vi "Untitled 1.vi"() -> ()   [LabVIEW 2025]
uses:
  <vilib>/LabVIEW Interface for Arduino/Type Defs/Pin Mode.ctl
  <vilib>/LabVIEW Interface for Arduino/LabVIEW Interface for Arduino.lvlib
panel:
  in  "stop":bool
  out "error out":errorcluster
  in  "Board":refnum<visa-resource-name>
  in  "Test cases":T1(ring)
  in  "Tab Control":T2(tab)
  in  "pin":u8
  in  "input val":u8
  out "Value":u8
  out "Outputs":bool[](array[boolean])
  in  "Set values":bool[](array[boolean])
  out "Voltage":dbl(knob) scale=0.0..5.0
  in  "Analog Input Pin (0)":u8
  out "Analog Port":dbl[](array[numeric])
  out "Waveform Chart":dbl(graph)
  in  "PWM 0 (0-255)":u8
  in  "PWM 1 (0-255)":u8
  in  "PWM 2 (0-255)":u8
  in  "PWM Pins":u8[](array[numeric])
  in  "Analog Input Pin":u8
  in  "pwm write single":u8
  in  "PWM Pin single":u8=3
  # "Arduino v4 tests"
  # "0x00 and 0x01 definitely work since every other case requires init and close to function"
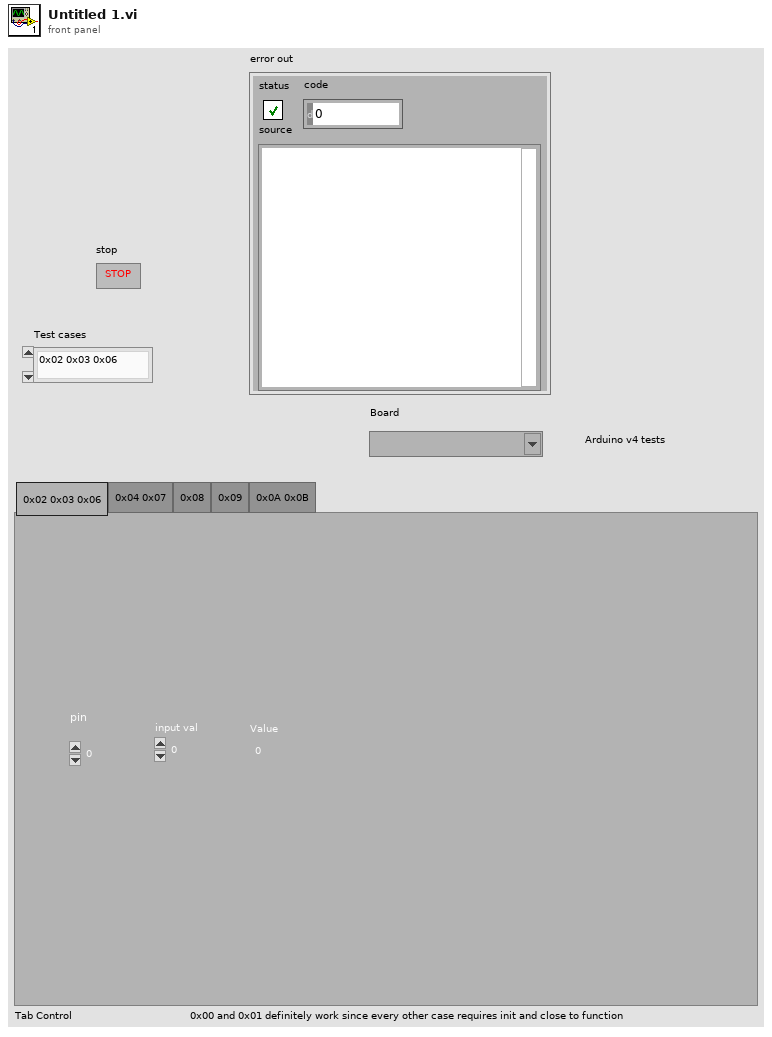
[diagram p1: front panel]
types:
  T1 = enum16{"0x02 0x03 0x06", "0x04 0x07", "0x08", "0x09", "0x0A 0x0B"}
  T2 = enum32{"0x02 0x03 0x06", "0x04 0x07", "0x08", "0x09", "0x0A 0x0B"}
  T3 = typedef "LabVIEW Interface for Arduino.lvlib/Pin Mode.ctl" = enum8{"Input", "Output"}
  T4 = typedef "LabVIEW Interface for Arduino.lvlib/Arduino Resource.ctl" = cluster{"VISA resource":refnum<visa-resource-name>, "Board Type":T5, "Connection Type":enum8{"USB / Serial"}, "Bytes Per Packet (15)":u8}
  T5 = typedef "LabVIEW Interface for Arduino.lvlib/Board Type.ctl" = enum16{"Uno", "Dimuelanove w/Atmega 328", "Mega 2560"}
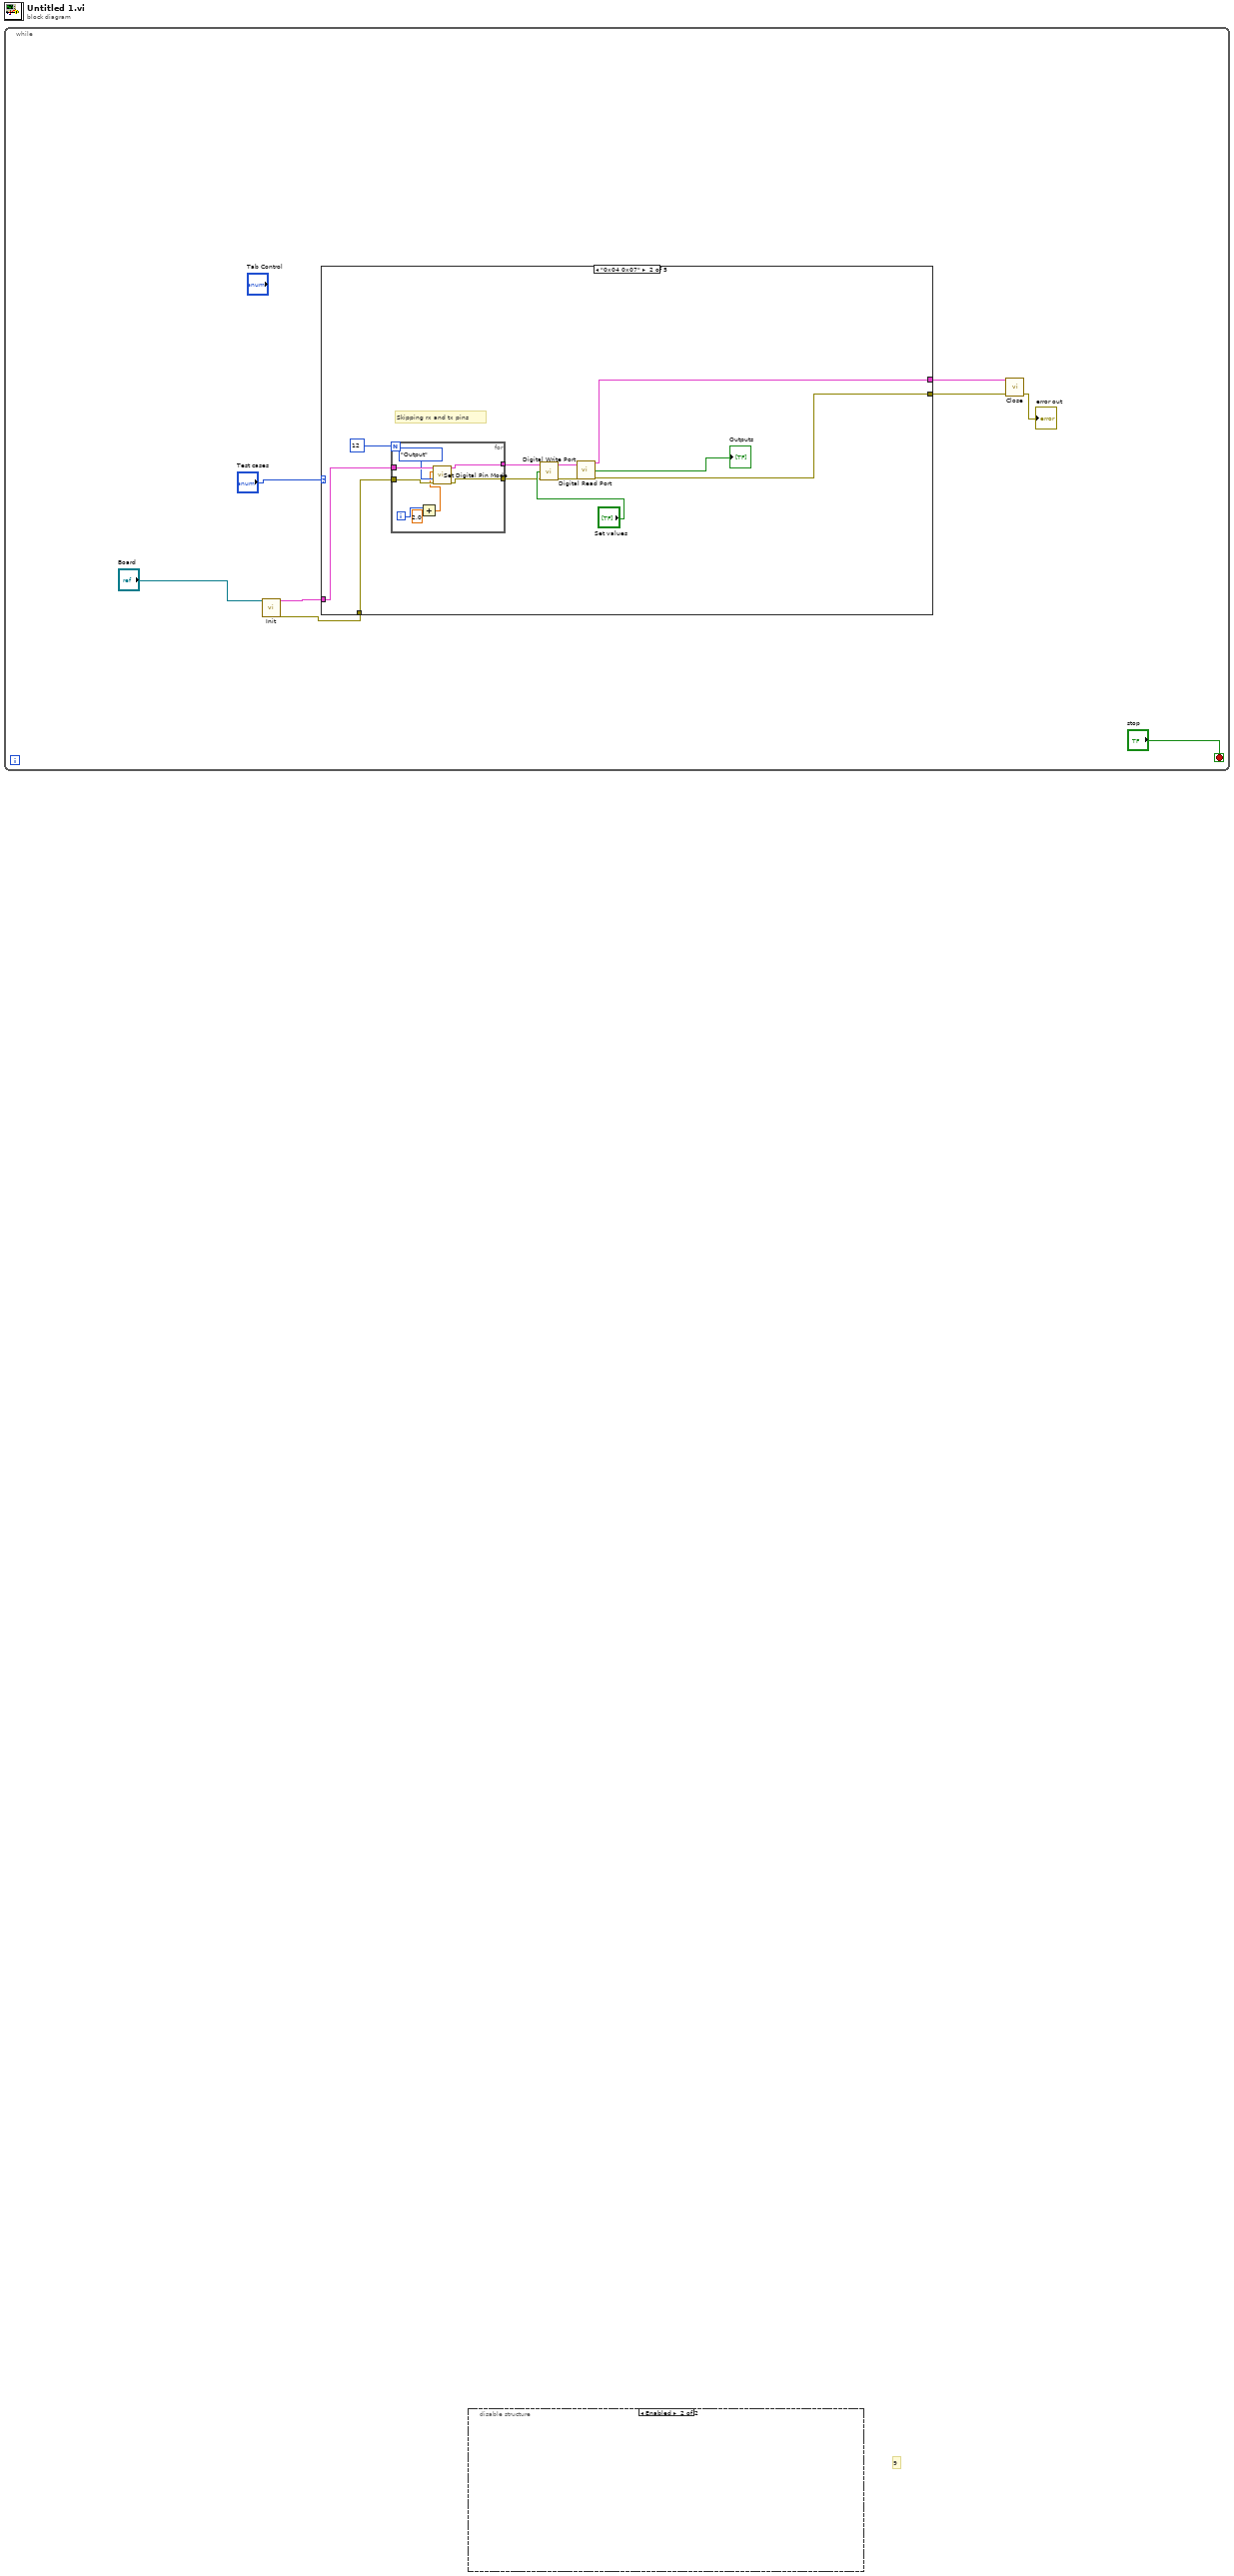
[diagram p0: block diagram]
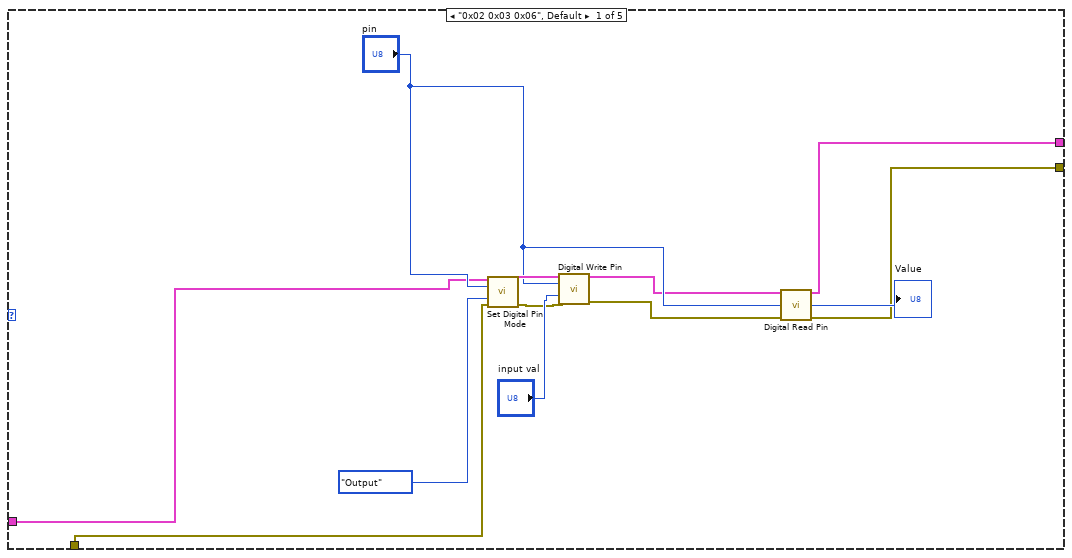
[diagram p2: hidden frame]
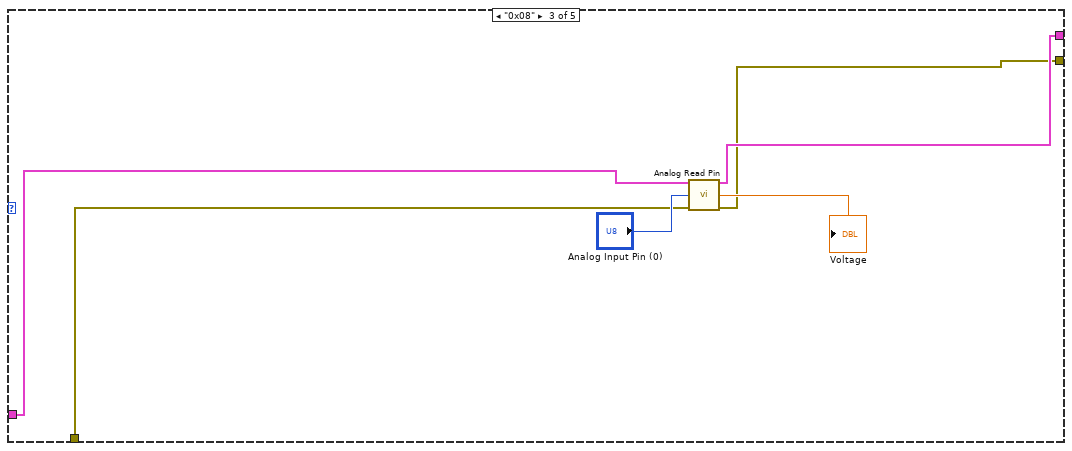
[diagram p3: hidden frame]
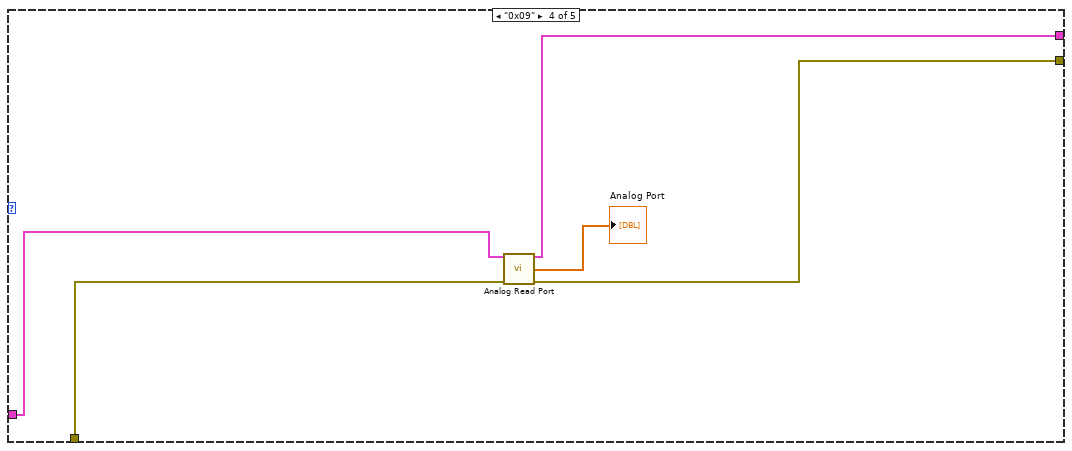
[diagram p4: hidden frame]
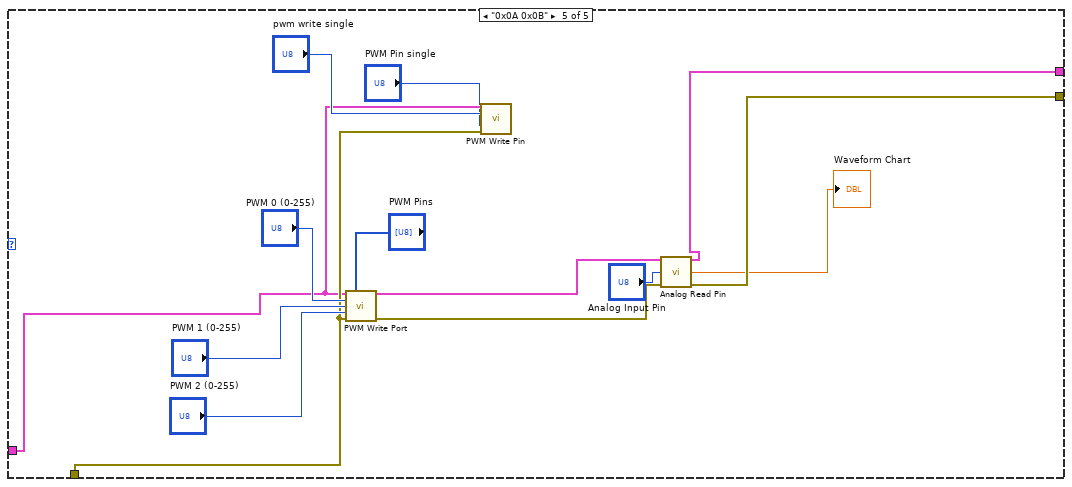
[diagram p5: hidden frame]
diagram:
  # "9"
  n1 = while {
    stop <- "stop" stop-if-true
    n2 = call <vilib>:"Init.vi"("VISA resource"="Board") -> ("Arduino Resource"=w6:T4, "error out"=w2:errorcluster)  [unwired: 17 in]
    n3 = case shown="\"0x04 0x07\"" "Test cases" {
      tunnel: w6 -> [w13 w24 w43 w48 w52]
      tunnel: [w12 w31 w42 w49 w57] -> w5
      tunnel: [w11 w28 w41 w46 w58] -> w4
      tunnel: w2 -> [w10 w25 w40 w47 w53]
      frame "0x02 0x03 0x06", Default {
        n4 = call <vilib>:"Set Digital Pin Mode.vi"("Arduino Resource"=w13, "Digital I/O Pin"="pin", "Pin Mode (Input)"=Pin_Mode."Output", "error in"=w10) -> ("Arduino Resource"=w18:T4, "error out"=w9:errorcluster)  [unwired: 10 in]
        n5 = call <vilib>:"Digital Write Pin.vi"("Arduino Resource"=w18, "Digital I/O Pin (0)"="pin", "Value (0)"="input val", "error in"=w9) -> ("Arduino Resource"=w15:T4, "error out"=w14:errorcluster)  [unwired: 10 in]
        n6 = call <vilib>:"Digital Read Pin.vi"("Arduino Resource"=w15, "Digital I/O Pin (0)"="pin", "error in"=w14) -> ("Arduino Resource"=w12:T4, "Value"=→"Value":u8, "error out"=w11:errorcluster)  [unwired: 10 in]
      }
      frame "0x04 0x07" {
        # "Skipping rx and tx pins"
        n7 = for {
          N: 12 -> [_]
          tunnel: w25 -> [w39]
          tunnel: w24 -> [w38]
          tunnel: [w36] -> w23
          tunnel: [w35] -> w22
          i -> [w33]
          n8 = Add(x=w33, y=2.0) -> (x+y=w32:dbl)
          n9 = call <vilib>:"Set Digital Pin Mode.vi"("Arduino Resource"=w38, "Digital I/O Pin"=w32, "Pin Mode (Input)"=Pin_Mode."Output", "error in"=w39) -> ("Arduino Resource"=w36:T4, "error out"=w35:errorcluster)  [unwired: 10 in]
        }
        n10 = call <vilib>:"Digital Write Port.vi"("Arduino Resource"=w23, "Pin Values"="Set values", "error in"=w22) -> ("Arduino Resource"=w27:T4, "error out"=w26:errorcluster)  [unwired: 11 in]
        n11 = call <vilib>:"Digital Read Port.vi"("Arduino Resource"=w27, "error in"=w26) -> ("Arduino Resource"=w31:T4, "Digital Port"=→"Outputs":bool[], "error out"=w28:errorcluster)  [unwired: 11 in]
      }
      frame "0x08" {
        n12 = call <vilib>:"Analog Read Pin.vi"("Arduino Resource"=w43, "Analog Input Pin (0)"="Analog Input Pin (0)", "error in"=w40) -> ("Arduino Resource"=w42:T4, "Voltage"=→"Voltage":dbl, "error out"=w41:errorcluster)  [unwired: 10 in]
      }
      frame "0x09" {
        n13 = call <vilib>:"Analog Read Port.vi"("Arduino Resource"=w48, "error in"=w47) -> ("Arduino Resource"=w49:T4, "Analog Port"=→"Analog Port":dbl[], "error out"=w46:errorcluster)  [unwired: 11 in]
      }
      frame "0x0A 0x0B" {
        n14 = call <vilib>:"PWM Write Port.vi"("Arduino Resource"=w52, "PWM Pins"="PWM Pins", "PWM 0 (0-255)"="PWM 0 (0-255)", "PWM 1 (0-255)"="PWM 1 (0-255)", "PWM 2 (0-255)"="PWM 2 (0-255)", "error in"=w53) -> ("Arduino Resource"=w60:T4, "error out"=w59:errorcluster)  [unwired: 7 in, 1 out]
        n15 = call <vilib>:"PWM Write Pin.vi"("Arduino Resource"=w52, "Duty Cycle (0 - 255)"="pwm write single", "PWM Pin (3)"="PWM Pin single", "error in"=w53) -> ()  [unwired: 10 in, 2 out]
        n16 = call <vilib>:"Analog Read Pin.vi"("Arduino Resource"=w60, "Analog Input Pin (0)"="Analog Input Pin", "error in"=w59) -> ("Arduino Resource"=w57:T4, "Voltage"=→"Waveform Chart":dbl, "error out"=w58:errorcluster)  [unwired: 10 in]
      }
    }
    n17 = call <vilib>:"Close.vi"("Arduino Resource"=w5, "error in"=w4) -> ("error out"=→"error out":errorcluster)  [unwired: 13 in]
  }
  n18 = disable-structure shown="Enabled" {
    frame Disabled {
    }
    frame Enabled {
    }
  }
